vi "RTEH Check Status.vi"(8 "Internal Status":cluster{"Status":T1, "Error Code":i32}) -> (0 "Internal Error":errorcluster, 3 "Skipped":bool)   [LabVIEW 2014]
uses:
  Controls/RTEH/RTEH Status Type.ctl
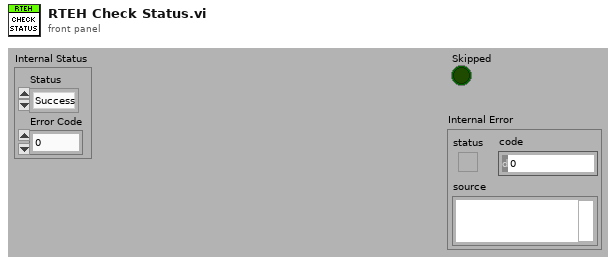
[diagram p1: front panel]
types:
  T1 = typedef "RTEH Status Type.ctl" = enum16{"Success", "Error", "Warning", "Skipped Notification"}
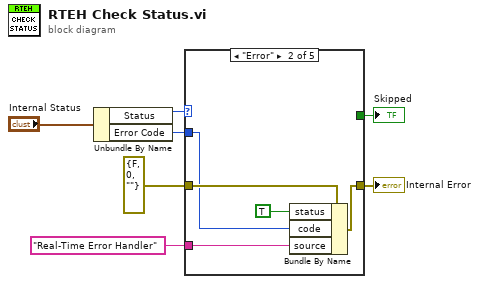
[diagram p0: block diagram]
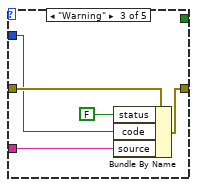
[diagram p3: hidden frame]
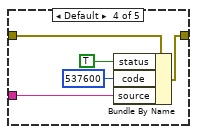
[diagram p4: hidden frame]
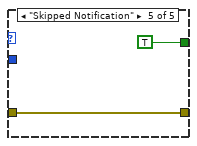
[diagram p5: hidden frame]
diagram:
  n1 = Unbundle By Name("Internal Status") -> ("Status"=w7:T1, "Error Code"=w4:i32)
  n2 = case shown="\"Error\"" w7 {
    tunnel: errorcluster {"status"=FALSE, "code"=0, "source"=""} ("Internal Error") -> [w8 w13 w18 w23 w25]
    tunnel: "Real-Time Error Handler" ("source") -> [_ w11 w16 w21 _]
    tunnel: w4 -> [_ w9 w14 _ _]
    tunnel: [w8 w12 w17 w22 w25] -> w3
    tunnel: [_ _ _ _ TRUE] -> w1
    frame "Success" {
    }
    frame "Error" {
      n3 = Bundle By Name(cluster=w13, "status"=TRUE, "code"=w9, "source"=w11) -> (w12:errorcluster)
    }
    frame "Warning" {
      n4 = Bundle By Name(cluster=w18, "status"=FALSE, "code"=w14, "source"=w16) -> (w17:errorcluster)
    }
    frame Default {
      n5 = Bundle By Name(cluster=w23, "status"=TRUE, "code"=537600, "source"=w21) -> (w22:errorcluster)
    }
    frame "Skipped Notification" {
    }
  }
  "Internal Error" <- w3
  "Skipped" <- w1
